vi "Cast To Variant (Array).vi"(8 "error in (no error)":errorcluster, 9 "datatype and defaults":variant, 11 "JSON Value in":refnum<class "JSON Value.lvclass">) -> (0 "error out":errorcluster, 2 "Variant":variant)   [LabVIEW 2016, in "JSFL Variant Support.lvlib"]
doc: "Populates a variant with the data contained in the given JSON instance. Valid types for datatype and defaults are: string, boolean, double, and a cluster of named controls of strings, booleans, doubles, or nested clusters.\n\nIf a given cluster contains values that aren't present in the JSON Object instance, the value in the datatype and defaults control is used instead and the defaulted keys output will contain the name of the path in the cluster to the control."
uses:
  JSFL Variant Support.lvlib
  JSON Value.lvclass
  Array/Index Array/Index Array (Value).vi
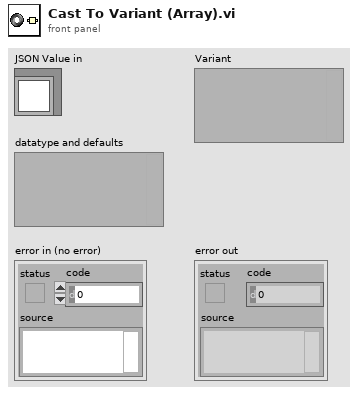
[diagram p1: front panel]
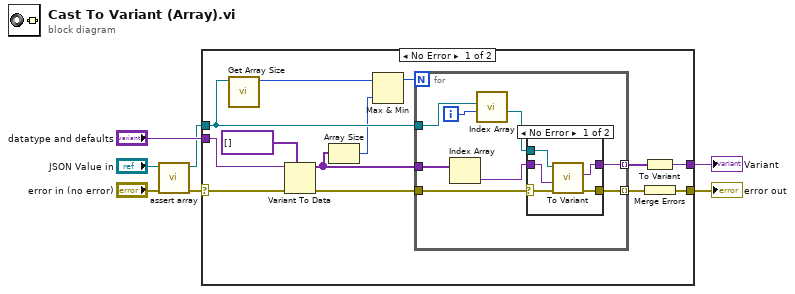
[diagram p0: block diagram]
diagram:
  n1 = call "assert array.vi"("error in (no error)"="error in (no error)", "JSON Value in"="JSON Value in") -> ("error out"=w3:errorcluster, "JSON Value out"=w1:refnum<class "JSON Value.lvclass">)  [unwired: 8 in]
  n2 = case shown="No Error" w3 {
    selector: w3 -> [w9 _]
    tunnel: [w20 _] -> w7
    tunnel: "datatype and defaults" -> [w19 _]
    tunnel: [w15 _] -> w4
    tunnel: w1 -> [w14 _]
    frame No Error {
      n3 = call "Get Array Size.vi"("JSON Value in"=w14) -> ("size(s)"=w11:i32)  [unwired: 9 in, 1 out]
      n4 = Variant To Data(error in=w9, type=variant[] [], Variant=w19) -> (data=w13:variant[], error out=w8:errorcluster)
      n5 = Array Size(array=w13) -> (size(s)=w12:i32)
      n6 = Max & Min(x=w11, y=w12) -> (max(x,y)=w10:i32)  [unwired: 1 out]
      n7 = for {
        N: w10 -> [_]
        tunnel: w13 -> [w23]
        tunnel: w14 -> [w28]
        tunnel: [w27] -> w17 mode=indexing
        tunnel: [w26] -> w16 mode=indexing
        tunnel: w8 -> [w25]
        i -> [w24]
        n8 = Index Array(array=w23) -> (element=w21:variant)  [unwired: 1 in]
        n9 = call-poly "Index Array.vi"("index"=w24, "JSON Value in"=w28) -> ("JSON Value out"=w22:refnum<class "JSON Value.lvclass">)  [unwired: 8 in, 1 out]
        n10 = case shown="No Error" w25 {
          selector: w25 -> [w29 w35]
          tunnel: w22 -> [w31 _]
          tunnel: [w32 w34] -> w27
          tunnel: [w30 w35] -> w26
          tunnel: w21 -> [w33 w34]
          frame No Error {
            n11 = call "To Variant.vi"("error in (no error)"=w29, "datatype and defaults"=w33, "JSON Value in"=w31) -> ("error out"=w30:errorcluster, "Variant"=w32:variant)  [unwired: 6 in, 1 out]
          }
          frame Error {
          }
        }
      }
      n12 = To Variant(anything=w17) -> (Variant=w20:variant)
      n13 = Merge Errors(w16) -> (w15:errorcluster)
    }
    frame Error {
    }
  }
  "error out" <- w4
  "Variant" <- w7
